vi "Wheel Control POS Brake.vi"(11 "Wheel DevRef In":T3={"Shooter Config reference"=refnum, "Shooter Data"={"MotorControlDevRef"={"DeviceStatus"={"status"=FALSE, "code"=0, "source"=""}, "Type"=enum."PWM", "PWM"={"PWM Channel"=enum."PWM 0", "DeadBand"={"Name"="", "maxPositivePwm"=0, "minPositivePwm"=0, "centerPwm"=0, "maxNegativePwm"=0, "minNegativePwm"=0, "angularRange"=0}}, "CAN"={"Device Number"=0, "SetOutput VI Ref"=variant(enum8{"Percent VBus", "Current", "Speed", "Position", "Voltage"} enum."Percent VBus"), "GetOutput VI Ref"=variant(refnum<k1> refnum), "Enable VI Ref"=variant(dbl 0.0), "Disable VI Ref"=variant(enum8{"Percent VBus", "Speed", "Position", "Slave", "Unchanged / Invalid", "Voltage Compensation", "Current", "Motion Profile"} enum."Percent VBus"), "Data"=variant}, "Invert"=FALSE}, "Set Point"=refnum, "Actual"=refnum}}) -> ()   [LabVIEW 2016, in "Wheel.lvlib"]
doc: "Help by FRC Team 836 - The RoboBees\n\nThis VI stops a wheel at the indicated postion using the tbh (Take Back Half) control VI."
uses:
  <userlib>/836-Library/Motion_Control/Shooter_Wheel/Wheel.lvlib
  <vilib>/Platform/TimedLoop/XDataNode/wakeup.ctl
  <vilib>/Platform/TimedLoop/XDataNode/XDNodeRunTimeDep.lvlib
  <vilib>/Platform/TimedLoop/XDataNode/nitl_modes.ctl
  <vilib>/Platform/TimedLoop/XDataNode/timing_clust.ctl
  <vilib>/platform/TimedLoop/XDataNode/XDataNode.xnode
  <vilib>/Rock Robotics/SystemInterfaces/DIO/FPGA_DIOPWMChannel.ctl
  <vilib>/Rock Robotics/WPI/PWM/WPI_PWMDeadband.ctl
  <vilib>/Rock Robotics/WPI/MotorControl/WPI_MotorControlDeviceRef.ctl
  <userlib>/836-Libraries/Motion_Control/Shooter_Wheel/Data.ctl
  <userlib>/836-Libraries/Motion_Control/Shooter_Wheel/Config.ctl
  <userlib>/836-Libraries/Motion_Control/Shooter_Wheel/WheelControl.ctl
  <vilib>/Rock Robotics/WPI/MotorControl/WPI_MotorControlType.ctl
  <vilib>/Rock Robotics/SystemInterfaces/Counter/FPGA_CounterCtrSystemIndex.ctl
  <vilib>/Rock Robotics/WPI/Counter/WPI_CounterDevRef.ctl
panel:
  in  "CounterDevRef in":T1={"DevStatus"={"status"=FALSE, "code"=0, "source"=""}, "CntIndex"=enum."Invalid"}
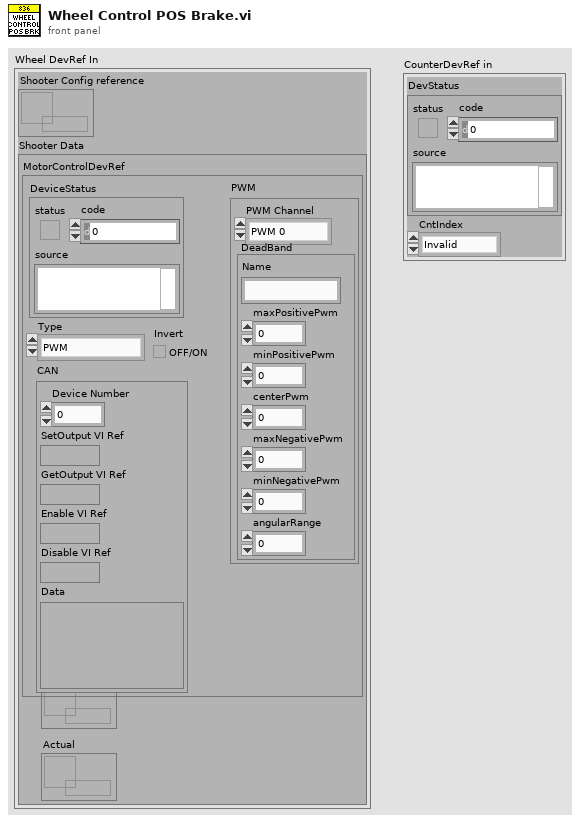
[diagram p1: front panel]
types:
  T1 = typedef "WPI_CounterDevRef.ctl" = cluster{"DevStatus":errorcluster, "CntIndex":T2}
  T2 = typedef "FPGA_CounterCtrSystemIndex.ctl" = enum8{"Ctr 0", "Ctr 1", "Ctr 2", "Ctr 3", "Ctr 4", "Ctr 5", "Ctr 6", "Ctr 7", "Invalid"}
  T3 = typedef "Wheel.lvlib/WheelControl.ctl" = cluster{"Shooter Config reference":refnum<data-value>, "Shooter Data":T4}
  T4 = typedef "Wheel.lvlib/Data.ctl" = cluster{"MotorControlDevRef":T5, "Set Point":refnum<k33>, "Actual":refnum<k33>}
  T5 = typedef "WPI_MotorControlDeviceRef.ctl" = cluster{"DeviceStatus":errorcluster, "Type":T6, "PWM":cluster{"PWM Channel":T7, "DeadBand":T8}, "CAN":cluster{"Device Number":u8, "SetOutput VI Ref":variant, "GetOutput VI Ref":variant, "Enable VI Ref":variant, "Disable VI Ref":variant, "Data":variant}, "Invert":bool}
  T6 = typedef "WPI_MotorControlType.ctl" = enum16{"PWM", "CAN"}
  T7 = typedef "FPGA_DIOPWMChannel.ctl" = enum8{"PWM 0", "PWM 1", "PWM 2", "PWM 3", "PWM 4", "PWM 5", "PWM 6", "PWM 7", "PWM 8", "PWM 9", "PWM MXP 0", "PWM MXP 1", "PWM MXP 2", "PWM MXP 3", "PWM MXP 4", "PWM MXP 5", "PWM MXP 6", "PWM MXP 7", "PWM MXP 8", "PWM MXP 9", "Invalid"}
  T8 = typedef "WPI_PWMDeadband.ctl" = cluster{"Name":string, "maxPositivePwm":i32, "minPositivePwm":i32, "centerPwm":i32, "maxNegativePwm":i32, "minNegativePwm":i32, "angularRange":u16}
  T9 = typedef "XDNodeRunTimeDep.lvlib/timing_clust.ctl" = cluster{"Expected End [f-1]":u64, "Actual End [f-1]":u64, "Finished Late? [f-1]":bool, "Expected End [i-1]":u64, "Actual End [i-1]":u64, "Finished Late? [i-1]":bool, "Expected Start [i]":u64, "Actual Start [i]":u64, "Expected Start [f]":u64, "Actual Start [f]":u64, "Source Name":string, "Structure Name":string, "Period":i64, "Deadline":i64, "Offset":i64, "Start":i64, "Priority":i32, "Timeout":i32, "Mode":T10, "Wakeup Reason":T11, "Error":errorcluster, "Source Type":string, "Secondary Source Type":string, "Global End Time":u64, "Global Start Time":u64, "Frame Duration":u64, "Iteration Duration":u64, "Assigned CPU":i32, "I/O Scan Engine Mode":u32}
  T10 = typedef "XDNodeRunTimeDep.lvlib/nitl_modes.ctl" = enum32{"No Change", "Process missed periods, maintain original phase", "Discard missed periods, maintain original phase", "Process missed periods, ignore original phase", "Discard missed periods, ignore original phase"}
  T11 = typedef "XDNodeRunTimeDep.lvlib/wakeup.ctl" = enum32{"Normal", "Aborted", "Asynchronous wakeup", "Timing source error", "Timed loop error", "Timeout"}
  T12 = typedef "Wheel.lvlib/Config.ctl" = cluster{"Period (ms)":i64, "TBH Gain":dbl, "Priority":i32, "PID gains":cluster{"proportional gain (Kc)":dbl, "integral time (Ti, min)":dbl, "derivative time (Td, min)":dbl}, "Stable (sec)":dbl, "Range":dbl}
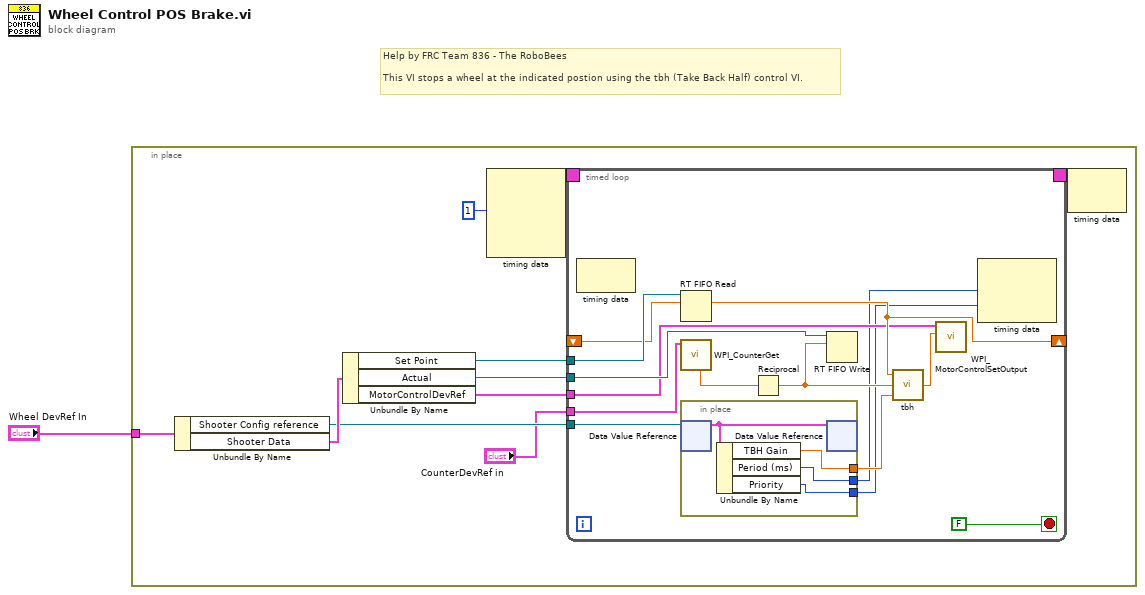
[diagram p0: block diagram]
diagram:
  # "Help by FRC Team 836 - The RoboBees\n\nThis VI stops a wheel at the indicated postion using the tbh (Take Back Half) control VI."
  n1 = in-place {
    in-place-border: "Wheel DevRef In" -> [w3]
    n2 = Unbundle By Name(w3) -> ("Shooter Config reference"=w4:refnum<data-value>, "Shooter Data"=w5:T4)
    n3 = Unbundle By Name(w5) -> ("Set Point"=w6:refnum<k33>, "Actual"=w7:refnum<k33>, "MotorControlDevRef"=w9:T5)
    n4 = node-c288(i64 1 ("Period")) -> (w11:T9)  [unwired: 3 in]
    n5 = timed-loop {
      timing: w11 -> [_]
      timing-out: [_] -> w10
      tunnel: w6 -> [w24]
      tunnel: w7 -> [w23]
      shift-right: [w21] -> _
      shift-left: _ -> [w22]
      tunnel: w9 -> [w19]
      tunnel: "CounterDevRef in" -> [w18]
      tunnel: w4 -> [w15]
      stop <- FALSE stop-if-true
      n6 = node-c288() -> ()  [unwired: 1 in, 1 out]
      n7 = RT FIFO Read(0:w24, 1:w22) -> (9:w21:dbl)  [unwired: 2 in, 4 out]
      n8 = call <vilib>:"WPI_CounterGet.vi"("CounterDevRef in"=w18) -> ("Period (sec)"=w17:dbl)  [unwired: 5 in, 5 out]
      n9 = in-place {
        in-place-border: [w29] -> w14
        in-place-border: [w28] -> w13
        in-place-border: [w27] -> w12
        n10 = in-place-dvr #1(w15) -> (w26:T12)  [unwired: 1 out]
        n11 = Unbundle By Name(w26) -> ("TBH Gain"=w29:dbl, "Period (ms)"=w28:i64, "Priority"=w27:i32)
        n12 = in-place-dvr #1(w26) -> ()  [unwired: 2 out]
      }
      n13 = Reciprocal(x=w17) -> (1/x=w16:dbl)
      n14 = RT FIFO Write(0:w23, 1:w16) -> ()  [unwired: 3 in, 4 out]
      n15 = call <userlib>:"tbh.vi"("Gain Factor"=w14, "Actual Value"=w16, "Desired Value"=w21) -> ("Out"=w20:dbl)
      n16 = call <vilib>:"WPI_MotorControlSetOutput.vi"("Output"=w20, "MotorControlDevRef"=w19) -> ()  [unwired: 7 in, 3 out]
      n17 = node-c288(w13, w12) -> ()  [unwired: 1 in, 1 out]
    }
    n18 = node-c288(w10) -> ()  [unwired: 1 out]
  }
